vi "Add_Item.vi"(8 "error constant 2":errorcluster, 11 "Database":T1[](array[typedef])) -> (0 "error constant":errorcluster, 3 "Modified Database":T1[](array[typedef]))   [LabVIEW 2022 SP3]
uses:
  Database_element.ctl
panel:
  in  "Cancel":bool
  in  "Add Item":bool
  out "Is input valid?":string
  in  "Input":T1
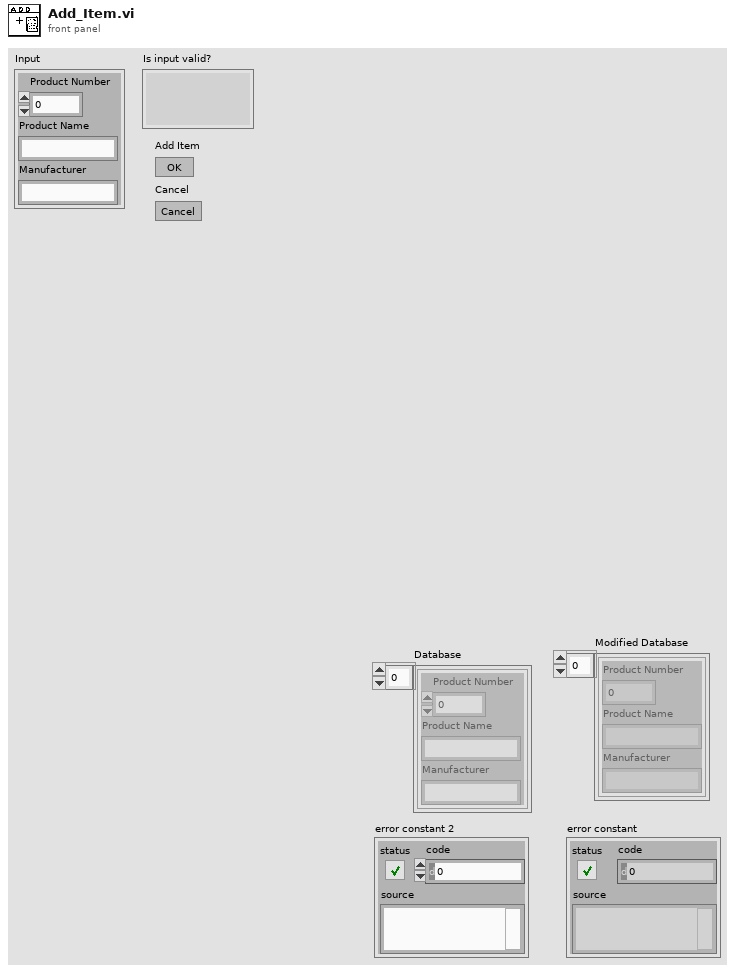
[diagram p1: front panel]
types:
  T1 = typedef "Database_element.ctl" = cluster{"Product Number":i32, "Product Name":string, "Manufacturer":string}
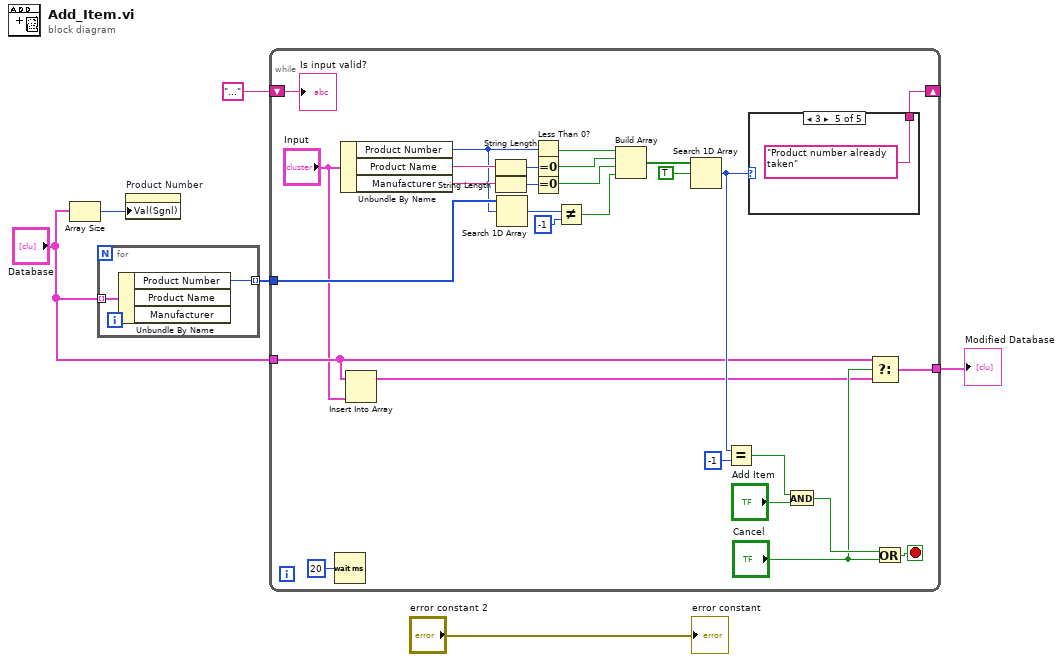
[diagram p0: block diagram]
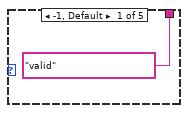
[diagram p2: hidden frame]
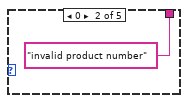
[diagram p3: hidden frame]
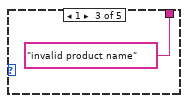
[diagram p4: hidden frame]
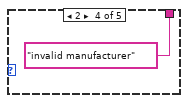
[diagram p5: hidden frame]
diagram:
  n1 = Array Size(array="Database") -> (size(s)=w4:i32)
  n2 = for {
    tunnel: "Database" -> [w8] mode=indexing
    tunnel: [w7] -> w3 mode=indexing
    n3 = Unbundle By Name(w8) -> ("Product Number"=w7:i32)  [unwired: 2 out]
  }
  n4 = property on="Product Number" class="DigNum (strict)"("Val(Sgnl)"=w4) -> ()  [unwired: 2 in, 2 out]
  n5 = while {
    shift-right: [w14] -> _
    shift-left: "..." -> [w34]
    tunnel: w3 -> [w26]
    tunnel: "Database" -> [w11]
    tunnel: [w12] -> w1
    stop <- w35 stop-if-true
    n6 = Wait (ms)(milliseconds to wait=u32 20) -> ()  [unwired: 1 out]
    n7 = Unbundle By Name("Input") -> ("Product Number"=w25:i32, "Product Name"=w33:string, "Manufacturer"=w32:string)
    n8 = Insert Into Array(array=w11, new element="Input") -> (w9:T1[])  [unwired: 1 in]
    n9 = String Length(string=w33) -> (length=w31:i32)
    n10 = String Length(string=w32) -> (length=w30:i32)
    n11 = Search 1D Array(1D array=w26, element=w25) -> (index of element=w24:i32)  [unwired: 1 in]
    n12 = Less Than 0?(x=w25) -> (x < 0?=w29:bool)
    n13 = Equal To 0?(x=w31) -> (x = 0?=w28:bool)
    n14 = Equal To 0?(x=w30) -> (x = 0?=w27:bool)
    n15 = Not Equal?(x=w24, y=-1) -> (x != y?=w22:bool)
    n16 = Build Array(w29, w28, w27, w22) -> (w20:bool[])
    n17 = Search 1D Array(1D array=w20, element=TRUE) -> (index of element=w18:i32)  [unwired: 1 in]
    n18 = Equal?(x=w18, y=-1) -> (x = y?=w17:bool)
    n19 = case shown="3" w18 {
      tunnel: ["valid" "invalid product number" "invalid product name" "invalid manufacturer" "Product number already taken"] -> w14
      frame -1, Default {
      }
      frame 0 {
      }
      frame 1 {
      }
      frame 2 {
      }
      frame 3 {
      }
    }
    n20 = And(x=w17, y="Add Item") -> (x .and. y?=w15:bool)
    n21 = Select(t=w11, s="Cancel", f=w9) -> (s? t:f=w12:T1[])
    n22 = Or(x=w15, y="Cancel") -> (x .or. y?=w35:bool)
    "Is input valid?" <- w34
  }
  "Modified Database" <- w1
  "error constant" <- "error constant 2"
